vi "Execute.vi"(8 "error in (no error)":errorcluster, 11 "CIFTemplatePlugin in":refnum<class "TemplatePlugin.lvclass">) -> (0 "error out":errorcluster, 3 "CIFTemplatePlugin out":refnum<class "TemplatePlugin.lvclass">)   [LabVIEW 2021, in "TemplatePlugin.lvclass"]
uses:
  TemplatePlugin.lvclass
  D:/dev/CIF-LVCore/src/CIFCore/Class/CIFCorePlugin.lvclass
  CIF-LVCore/src/CIFCore/Class/CIFCorePlugin.lvclass/CIFCorePlugin.ctl
  CIF-LVCore/src/CIFCore/Class/Typedef/Energized States.ctl
  TemplatePlugin.lvclass/TemplatePlugin.ctl
  CIF-LVCore/src/Channels/CIFChannelMng/CIFChannelMng.lvclass/CIFChannelMng.ctl
  <vilib>/CIF Foundation/CIF Channels Core/CIFChannels/CIFChannels.lvclass/CIFChannels.ctl
  <vilib>/CIF Foundation/CIF Channels Core/CIF_NIChn/Double/CIF_NIChn_Double.lvclass/CIF_NIChn_Double.ctl
  <vilib>/CIF Foundation/CIF Channels Core/CIF_NIChn/NIChn/CIF_NIChn.lvclass/CIF_NIChn.ctl
  <vilib>/CIF Foundation/CIF Channels Core/CIF_NIChn/U64/CIF_NIChn_U64.lvclass/CIF_NIChn_U64.ctl
  <vilib>/CIF Foundation/CIF Utilities/Time/System Time/Get System Time.vi
  CIF-LVCore/src/CIFCore/Class/Accessors/Timestamps/Write Execute TS.vi
  <vilib>/Utility/error.llb/Clear Errors.vi
  <vilib>/CIF Foundation/CIF Utilities/Time/System Time/Sleep Until Future Time.vi
  CIF-LVCore/src/CIFCore/Class/Accessors/Read Sleep Limits (ns).vi
  CIF-LVCore/src/CIFCore/Class/Accessors/Timestamps/Write Target Wake TS.vi
  CIF-LVCore/src/CIFCore/Class/SubVIs/Start Running.vi
  CIF-LVCore/src/CIFCore/Common/Utilities/Add Error.vi
  CIF-LVCore/src/CIFCore/Class/Accessors/Read Plugin Name.vi
  CIF-LVCore/src/CIFCore/Class/Accessors/Timestamps/Read Running TS.vi
  CIF-LVCore/src/CIFCore/Class/Accessors/Read Running Internal Data.vi
  CIF-LVCore/src/CIFCore/Class/Accessors/Read Timing Override.vi
  CIF-LVCore/src/CIFCore/Class/Accessors/Read Common Config.vi
  <vilib>/CIF Foundation/CIF Channels Core/CIF_NIChn/Double/Core/Read Double Direct Dispatch.vi
  <vilib>/CIF Foundation/CIF Channels Core/CIF_NIChn/U64/Core/Read U64 Direct Dispatch.vi
  <vilib>/CIF Foundation/CIF Channels Core/CIF_NIChn/Double/Core/Write Double Direct Dispatch.vi
  <vilib>/CIF Foundation/CIF Channels Core/CIF_NIChn/U64/Core/Write U64 Direct Dispatch.vi
  CIF-LVCore/src/CIFCore/Class/Accessors/Read Channel Array.vi
  CIF-LVCore/src/CIFCore/Class/Accessors/Write Channel Array.vi
  CIF-LVCore/src/CIFCore/Class/Accessors/Monitor/Write Double 1.vi
  CIF-LVCore/src/CIFCore/Class/Accessors/Monitor/Write U64 1.vi
  CIF-LVCore/src/CIFCore/Class/Accessors/Monitor/Write I64 1.vi
  CIF-LVCore/src/CIFCore/Class/Accessors/Monitor/Write I64 2.vi
  <vilib>/CIF Foundation/CIF Utilities/Time/System Time/LabVIEW Time to TAI Time.vi
  <vilib>/CIF Foundation/CIF Utilities/Time/SubVIs/Add Error.vi
  <vilib>/CIF Foundation/CIF Utilities/Errors/Append Error Location.vi
  <vilib>/CIF Foundation/CIF Channels Core/CIF_NIChn/NIChn/Accessors/Read CIF Channel.vi
  <vilib>/CIF Foundation/CIF Channels Core/CIF_NIChn/NIChn/SubVIs/Check Disconnect.vi
  <vilib>/CIF Foundation/CIF Channels Core/CIF_NIChn/Double/Core/Read Double Direct Dispatch.vi/d7866fd0-95aa-4020-8d43-a7942dcd60c7.vi
  <vilib>/CIF Foundation/CIF Channels Core/CIF_NIChn/NIChn/Accessors/Write CIF Channel.vi
  <vilib>/CIF Foundation/CIF Channels Core/CIFChannels/Accessors/Read Channel State.vi
  <vilib>/CIF Foundation/CIF Channels Core/CIFChannels/Accessors/Read Direction.vi
  <vilib>/CIF Foundation/CIF Channels Core/CIFChannels/Accessors/Read Tag Forced.vi
  <vilib>/CIF Foundation/CIF Channels Core/CIF_NIChn/U64/Core/Read U64 Direct Dispatch.vi/710841dd-0ab1-4cc4-9fc9-38c3cb3ebca4.vi
  <vilib>/CIF Foundation/CIF Channels Core/CIF_NIChn/Double/Core/Write Double Direct Dispatch.vi/3ad77888-3ad1-44f6-bae2-ae7fcd897aae.vi
  <vilib>/CIF Foundation/CIF Channels Core/CIF_NIChn/U64/Core/Write U64 Direct Dispatch.vi/730631e7-244d-420d-bc5d-6871287ea090.vi
  CIF-LVCore/src/Channels/CIFChannelMng/Accessors/Read Channel Array.vi
  CIF-LVCore/src/Channels/CIFChannelMng/Accessors/Write Channel Array.vi
  <vilib>/CIF Foundation/CIF Channels Core/CIFChannels/Accessors/Write Channel State.vi
  <vilib>/CIF Foundation/CIF Channels Core/CIFChannels/Accessors/Read Tag Disconnect Behavior.vi
  <vilib>/CIF Foundation/CIF Channels Core/CIF_NIChn/Double/Core/Read Double Direct Dispatch.vi/d7866fd0-95aa-4020-8d43-a7942dcd60c7.vi/c28b0ead-42ad-4072-80a2-aca7f2bd7ce3.vi
  <vilib>/CIF Foundation/CIF Channels Core/CIF_NIChn/Double/Core/Read Double Direct Dispatch.vi/d7866fd0-95aa-4020-8d43-a7942dcd60c7.vi/219d0231-d98b-4193-b5cc-84f90e3c9091.vi
  <vilib>/CIF Foundation/NI Channels/SubVIs/Get dll Path.vi
  <vilib>/CIF Foundation/CIF Channels Core/CIF_NIChn/U64/Core/Read U64 Direct Dispatch.vi/710841dd-0ab1-4cc4-9fc9-38c3cb3ebca4.vi/c28b0ead-42ad-4072-80a2-aca7f2bd7ce3.vi
  <vilib>/CIF Foundation/CIF Channels Core/CIF_NIChn/U64/Core/Read U64 Direct Dispatch.vi/710841dd-0ab1-4cc4-9fc9-38c3cb3ebca4.vi/219d0231-d98b-4193-b5cc-84f90e3c9091.vi
  <vilib>/CIF Foundation/CIF Channels Core/CIF_NIChn/Double/Core/Write Double Direct Dispatch.vi/3ad77888-3ad1-44f6-bae2-ae7fcd897aae.vi/4bc1c15b-36ab-481f-b8dd-c64075ce723a.vi
  <vilib>/CIF Foundation/CIF Channels Core/CIF_NIChn/Double/Core/Write Double Direct Dispatch.vi/3ad77888-3ad1-44f6-bae2-ae7fcd897aae.vi/d83cb72b-7713-41fc-a3d1-682de79cf574.vi
  <vilib>/CIF Foundation/CIF Channels Core/CIF_NIChn/U64/Core/Write U64 Direct Dispatch.vi/730631e7-244d-420d-bc5d-6871287ea090.vi/4bc1c15b-36ab-481f-b8dd-c64075ce723a.vi
  <vilib>/CIF Foundation/CIF Channels Core/CIF_NIChn/U64/Core/Write U64 Direct Dispatch.vi/730631e7-244d-420d-bc5d-6871287ea090.vi/d83cb72b-7713-41fc-a3d1-682de79cf574.vi
  <vilib>/CIF Foundation/CIF Channels Core/CIF_NIChn/Double/CIF_NIChn_Double.lvclass
  C:/Program Files/National Instruments/LabVIEW 2021/vi.lib/CIF Foundation/CIF Channels Core/CIFChannels/CIFChannels.lvclass
  C:/Program Files/National Instruments/LabVIEW 2021/vi.lib/CIF Foundation/CIF Channels Core/CIF_NIChn/NIChn/CIF_NIChn.lvclass
  <vilib>/CIF Foundation/CIF Channels Core/CIF_NIChn/NIChn/CIF_NIChn.lvclass
  <vilib>/CIF Foundation/CIF Channels Core/CIF_NIChn/U64/CIF_NIChn_U64.lvclass
  <vilib>/CIF Foundation/CIF Channels Core/CIFChannels/CIFChannels.lvclass
  CIF-LVCore/src/CIFCore/Class/CIFCorePlugin.lvclass
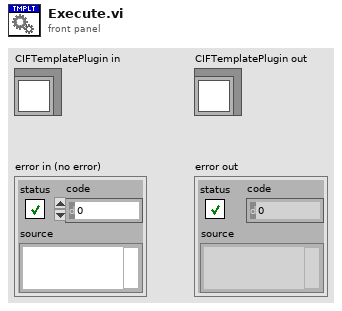
[diagram p1: front panel]
types:
  T1 = typedef "CIFCorePlugin.lvclass/Energized States.ctl" = enum16{"Listen", "Prepare", "Execute", "Housekeep", "Cleanup", "Destroy"}
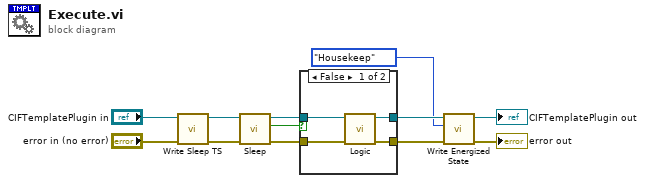
[diagram p0: block diagram]
diagram:
  n1 = call "Write Sleep TS.vi"("error in (no error)"="error in (no error)", "CIFCorePlugin in"="CIFTemplatePlugin in") -> ("error out"=w8:errorcluster, "CIFCorePlugin out"=w9:refnum<class "TemplatePlugin.lvclass">)  [unwired: 8 in]
  n2 = call "Sleep.vi"("error in (no error)"=w8, "CIFCorePlugin in"=w9) -> ("error out"=w10:errorcluster, "Housekeep only"=w7:bool, "CIFCorePlugin out"=w11:refnum<class "TemplatePlugin.lvclass">)  [unwired: 7 in]
  n3 = case shown="False" w7 {
    tunnel: [w13 w17] -> w2
    tunnel: [w14 w18] -> w5
    tunnel: w11 -> [w15 w18]
    tunnel: w10 -> [w16 w17]
    frame False {
      n4 = call "Logic.vi"("error in (no error)"=w16, "CIFTemplatePlugin in"=w15) -> ("error out"=w13:errorcluster, "CIFTemplatePlugin out"=w14:refnum<class "TemplatePlugin.lvclass">)  [unwired: 8 in]
    }
    frame True {
    }
  }
  n5 = call "Write Energized State.vi"("error in (no error)"=w2, "Energized State"=Energized_States."Housekeep", "CIFCorePlugin in"=w5) -> ("error out"=→"error out":errorcluster, "CIFCorePlugin out"=→"CIFTemplatePlugin out":refnum<class "TemplatePlugin.lvclass">)  [unwired: 7 in]
